vi "Set Reader Model.vi"(0 "COM":refnum<visa-resource-name>, 1 "Timeout (ms)":u32=500, 5 "Data":string(combo)="A", 7 "Address":string="01", 11 "error in (no error)":errorcluster) -> (4 "COM OUT":refnum<visa-resource-name>, 6 "ReceiveString":string, 15 "error out":errorcluster)   [LabVIEW 2020, in "Reader.lvlib"]
uses:
  Reader.lvlib
  b4065710-9efc-474a-baa2-b12afd0568aa.vi
panel:
  # "A指令读取模式\nB直接模式\nC外部触发模式"
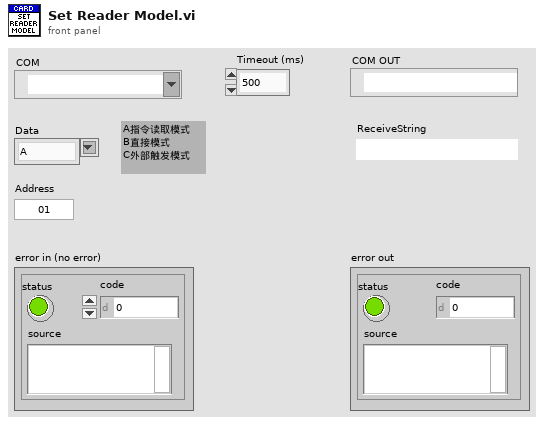
[diagram p1: front panel]
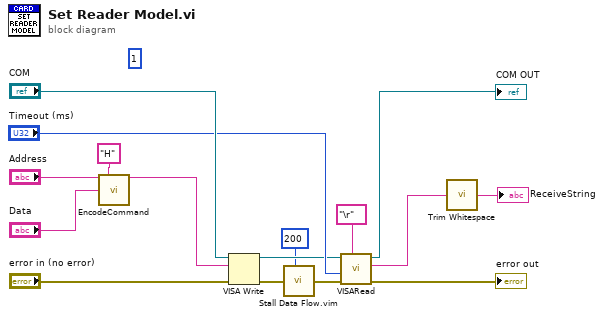
[diagram p0: block diagram]
diagram:
  (unwired) 1
  n1 = call "EncodeCommand.vi"("Address"="Address", "Function"="H", "Data"="Data") -> ("Command String"=w13:string)  [unwired: 11 in, 1 out]
  n2 = VISA Write(VISA resource name="COM", write buffer=w13, error in (no error)="error in (no error)") -> (VISA resource name out=w7:refnum<visa-resource-name>, error out=w6:errorcluster)  [unwired: 1 out]
  n3 = call "Stall Data Flow.vim"("value in"=w6, "milliseconds to wait"=u32 200) -> ("value out"=w2:errorcluster)  [unwired: 1 out]
  n4 = call "VISARead.vi"("Termination Char (blank)"="\r" ("Read regular"), "error in (no error)"=w2, "Timeout (ms)"="Timeout (ms)", "Resource in"=w7) -> ("error out"=→"error out":errorcluster, "Read Char"=w4:string, "Resource out"=→"COM OUT":refnum<visa-resource-name>)  [unwired: 5 in]
  n5 = call <vilib>:"Trim Whitespace.vi"("string"=w4) -> ("trimmed string"=→"ReceiveString":string)  [unwired: 1 in]
